vi "Write Scan.vi"(6 "Scan number":i32, 8 "error in":errorcluster, 9 "Data channels":waveform(dbl)[](array[waveform]), 10 "Data channel names":string[](array[string]), 11 "tdms file in":refnum<k34>) -> (0 "error out":errorcluster, 3 "tdms file out":refnum<k34>)   [LabVIEW 2021]
panel:
  # "V"
  # "I"
  # "dIdV"
  # "T"
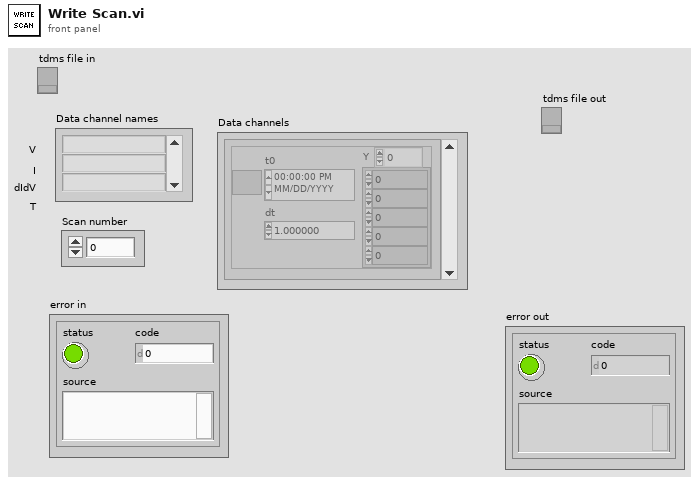
[diagram p1: front panel]
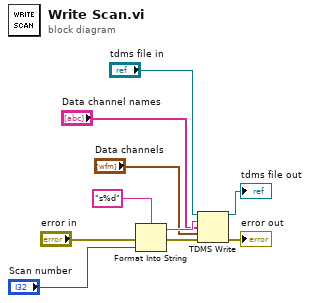
[diagram p0: block diagram]
diagram:
  n1 = Format Into String(format string="s%d", error in="error in", "Scan number") -> (resulting string=w10:string, error out=w8:errorcluster)  [unwired: 1 in]
  n2 = TDMS Write(0:"tdms file in", 5:w10, 7:"Data channel names", 9:"Data channels", 11:w8) -> (4:→"tdms file out":refnum<k34>, 15:→"error out":errorcluster)  [unwired: 1 in, 2 out]
